vi "Coord window-Save.vi"(11 "file path":path) -> (0 "error out":errorcluster)   [LabVIEW 2020]
uses:
  Globals/Coord window-Globals.vi
  <userlib>/My Palettes.lib/Files & paths/Spreadsheet/Write To Spreadsheet File (string)-Mod.vi
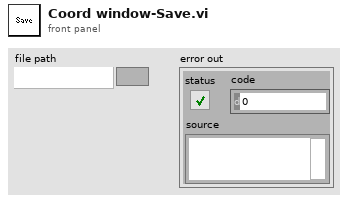
[diagram p1: front panel]
types:
  T1 = typedef "Coordinate list window refs.ctl" = cluster{"Window Name (i.e. Key)":string, "menu reference":refnum<k9>, "VI's reference":refnum<vi>, "Pane 1":refnum<vi>, "Pane 2":refnum<vi>, "Coord Listbox":refnum<vi>, "File name":refnum<vi>, "Picture Map":refnum<vi>, "Stage XYZ Position ind.":refnum<vi>}
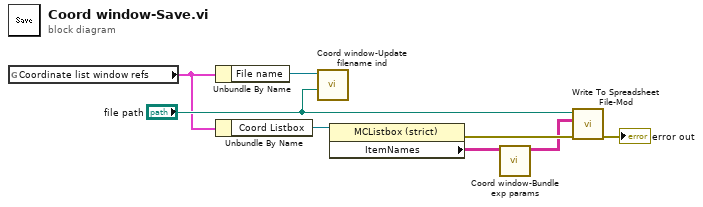
[diagram p0: block diagram]
diagram:
  n1 = global read "Coord window-Globals.vi" "Coordinate list window refs"() -> (w3:T1)
  n2 = Unbundle By Name(w3) -> ("File name"=w7:refnum<vi>)
  n3 = Unbundle By Name(w3) -> ("Coord Listbox"=w6:refnum<vi>)
  n4 = call "Coord window-Update filename ind.vi"("File path"="file path", "File name indicator ref"=w7) -> ()  [unwired: 9 in, 1 out]
  n5 = property on="Property Node" class="MCListbox (strict)"(reference=w6) -> (error out=w5:errorcluster, "ItemNames"=w2:string[][])  [unwired: 1 in, 1 out]
  n6 = call "Coord window-Bundle exp params.vi"("Item Names"=w2) -> ("Item Names + exp params"=w1:string[][])  [unwired: 10 in]
  n7 = call-poly <userlib>:"Write To Spreadsheet File-Mod.vi"("error in"=w5, "2D data"=w1, "file path (dialog if empty)"="file path") -> ("error out"=→"error out":errorcluster)  [unwired: 7 in, 1 out]
